vi "determine_harmonics.vi"(0 "FFT magnitude":cluster{"f0":dbl, "df":dbl, "magnitude":dbl[]}={"f0"=0.0, "df"=71.42857142857356, "magnitude"=array[7000 elements]}, 1 "FFT phase":cluster{"f0":dbl, "df":dbl, "phase":dbl[]}={"f0"=0.0, "df"=71.42857142857356, "phase"=array[7000 elements]}, 3 "TxRxParams":T1={"sample rate"=1000000.0, "Transmit frequency"=25000.0, "Transmit amplitude"=1.577, "sample rate digital out"=40000.0, "TX cycles"=600, "sample rate DAQ1"=1000000.0, "Receive frequency"=75000.0, "Receive range"=1.0, "TX harmonics"=[50000.0, 75000.0, 100000.0, 125000.0, 150000.0, 175000.0, 200000.0, 225000.0]} {"TX harmonics" format="%#_6p"; "Receive frequency" format="%#_6p"; "sample rate DAQ1" format="%#_6p"; "sample rate digital out" format="%#_6p"; "Transmit frequency" format="%#_6p"; "sample rate" format="%#_6p"}, 4 "TX harmonics mag baseline":dbl[](array[numeric])=[0.0, 0.0, 0.0, 0.0, 0.0, 0.0, 0.0, 0.0, 0.0, 0.0, 0.0], 5 "TX harmonics  phase baseline":dbl[](array[numeric])=[0.0, 0.0, 0.0, 0.0, 0.0, 0.0, 0.0, 0.0, 0.0, 0.0, 0.0], 6 "baseline phase":dbl, 7 "baseline magnitude":dbl) -> (12 "f0 phase":dbl=1.9394134400610221, 13 "f0 mag":dbl=0.024822285377457173, 14 "RX magnitude":dbl=0.0015696795969549263, 15 "RX phase":dbl=0.51499599210196, 17 "F3/F2":dbl, 18 "mag f2-f9":dbl[](array[numeric])=[0.07635364629802971, 0.0015696795969549263, 2.5850938198280388e-05, 3.5062095809530066e-05, 2.655041530081199e-05, 3.019279214108981e-05, 1.4173746366290001e-05, 4.367321701979328e-05], 19 "phase f2-f9":dbl[](array[numeric])=[2.093173382122955, 0.51499599210196, -2.573476238721069, 0.1764472036180968, -2.656638672525607, 2.555905242708201, -1.1093217629525705, -0.18697146017335703])   [LabVIEW 2021]
panel:
  out "TX harmonics":dbl[](array[numeric])=[50000.0, 75000.0, 100000.0, 125000.0, 150000.0, 175000.0, 200000.0, 225000.0] format="%#_6p"
  out "RxFreq":dbl=75000.0 format="%#_13g"
  out "TxFreq":dbl=25000.0 format="%#_13g"
  # "Inputs:"
  # "Keep default baseline value under all circumstances zero!!!!"
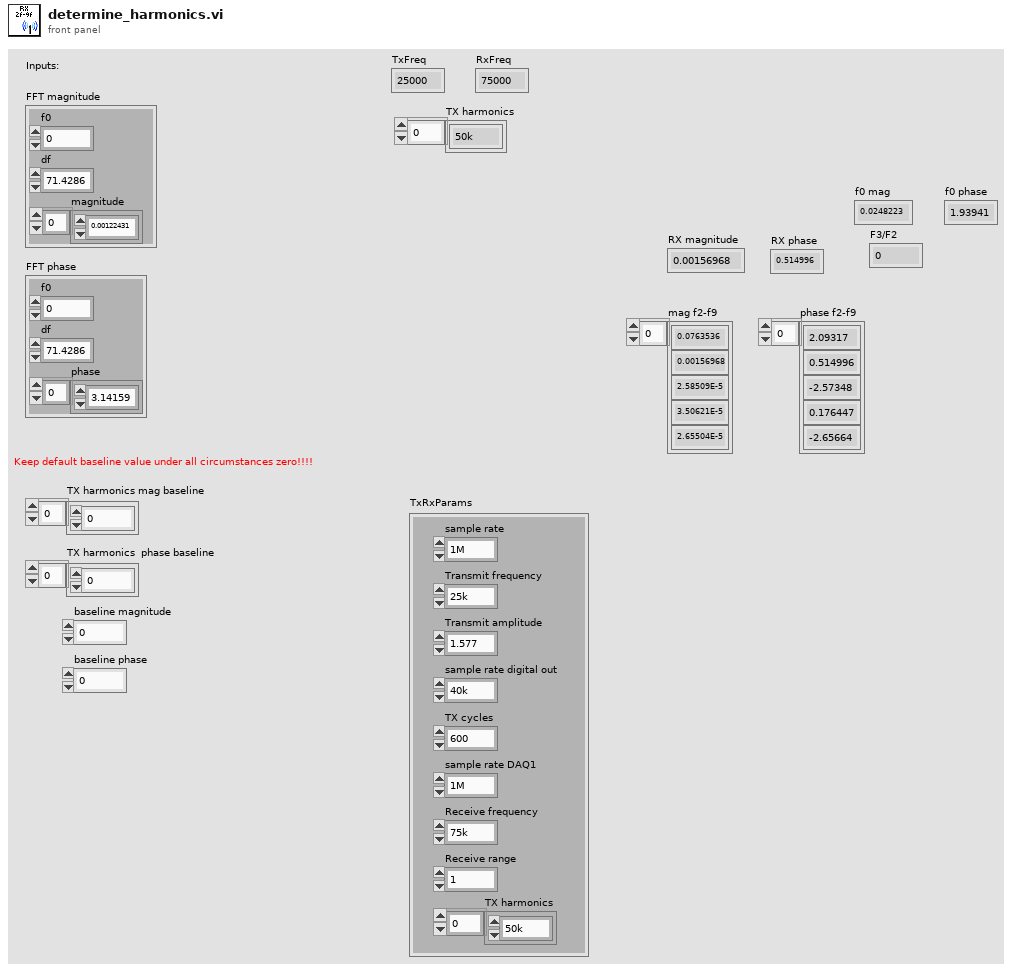
[diagram p1: front panel]
types:
  T1 = cluster{"sample rate":dbl, "Transmit frequency":dbl, "Transmit amplitude":dbl, "sample rate digital out":dbl, "TX cycles":i32, "sample rate DAQ1":dbl, "Receive frequency":dbl, "Receive range":dbl, "TX harmonics":dbl[]}
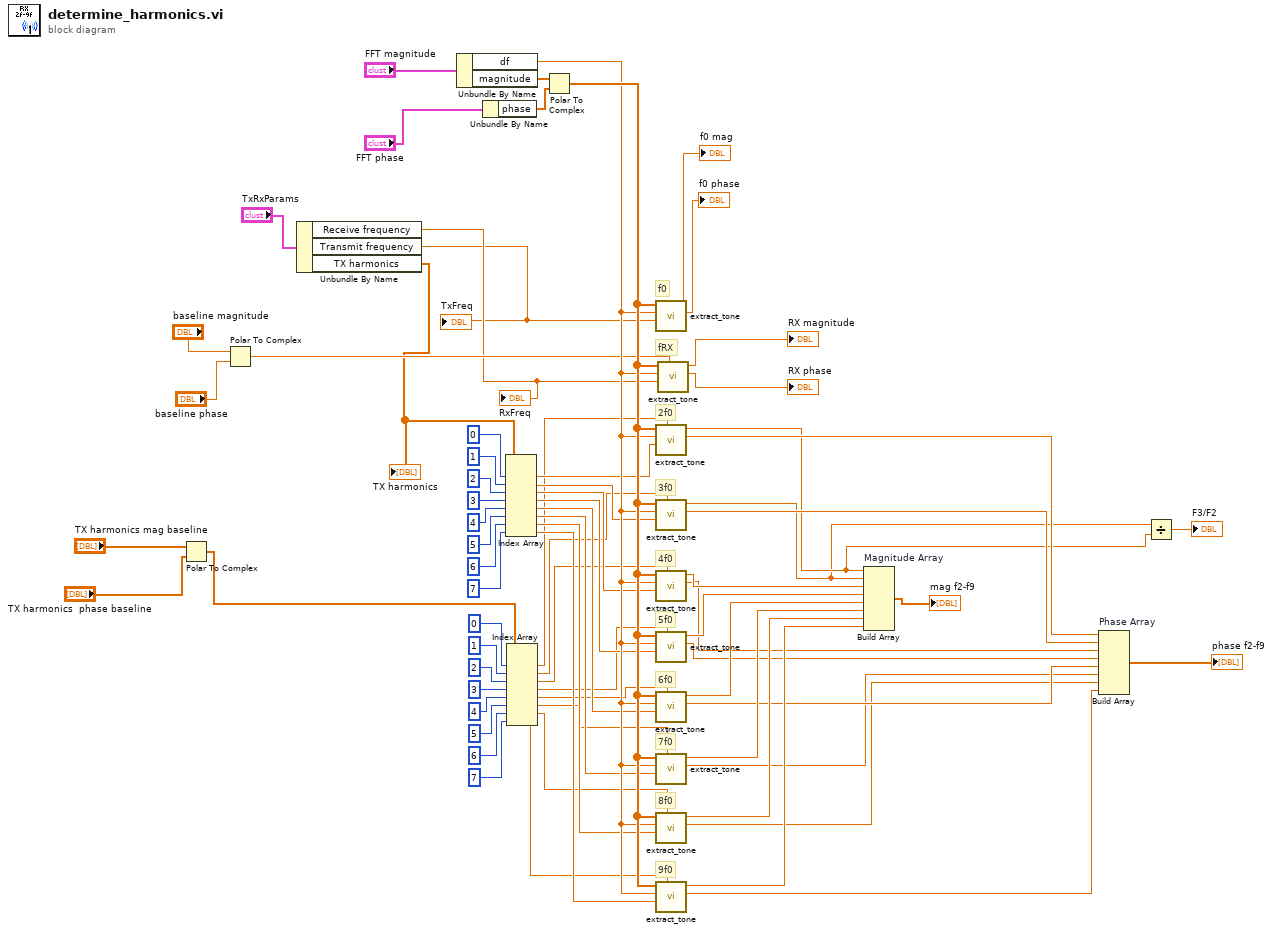
[diagram p0: block diagram]
diagram:
  # "fRX"
  # "9f0"
  # "8f0"
  # "7f0"
  # "6f0"
  # "5f0"
  # "4f0"
  # "3f0"
  # "2f0"
  # "f0"
  n1 = Polar To Complex(1:"TX harmonics  phase baseline", 2:"TX harmonics mag baseline") -> (0:w16:cdb[])
  n2 = Polar To Complex(1:"baseline phase", 2:"baseline magnitude") -> (0:w28:cdb)
  n3 = Unbundle By Name("TxRxParams") -> ("Receive frequency"=w6:dbl, "Transmit frequency"=w5:dbl, "TX harmonics"=w4:dbl[])
  "TxFreq" <- w5
  "RxFreq" <- w6
  "TX harmonics" <- w4
  n4 = Unbundle By Name("FFT magnitude") -> ("df"=w45:dbl, "magnitude"=w69:dbl[])
  n5 = Unbundle By Name("FFT phase") -> ("phase"=w68:dbl[])
  n6 = Index Array(array=w4, index #1=0 ("index"), index #2=1 ("index"), index #3=2 ("index"), index #4=3 ("index"), index #5=4 ("index"), index #6=5 ("index"), index #7=6 ("index"), index #8=7 ("index")) -> (element #1=w44:dbl, element #2=w35:dbl, element #3=w34:dbl, element #4=w33:dbl, element #5=w32:dbl, element #6=w31:dbl, element #7=w30:dbl, element #8=w29:dbl)
  n7 = Index Array(array=w16, index #1=0 ("index"), index #2=1 ("index"), index #3=2 ("index"), index #4=3 ("index"), index #5=4 ("index"), index #6=5 ("index"), index #7=6 ("index"), index #8=7 ("index")) -> (element #1=w15:cdb, element #2=w14:cdb, element #3=w13:cdb, element #4=w12:cdb, element #5=w11:cdb, element #6=w10:cdb, element #7=w9:cdb, element #8=w8:cdb)
  n8 = Polar To Complex(1:w68, 2:w69) -> (0:w46:cdb[])
  n9 = call "extract_tone.vi"("tone frequency [Hz]"=w5, "df"=w45, "complex fft"=w46) -> ("phase (rad)"=→"f0 phase":dbl, "amplitude"=→"f0 mag":dbl)  [unwired: 7 in]
  n10 = call "extract_tone.vi"("complex baseline"=w15, "tone frequency [Hz]"=w44, "df"=w45, "complex fft"=w46) -> ("phase (rad)"=w59:dbl, "amplitude"=w3:dbl)  [unwired: 6 in]
  n11 = call "extract_tone.vi"("complex baseline"=w14, "tone frequency [Hz]"=w35, "df"=w45, "complex fft"=w46) -> ("phase (rad)"=w50:dbl, "amplitude"=w2:dbl)  [unwired: 6 in]
  n12 = call "extract_tone.vi"("complex baseline"=w13, "tone frequency [Hz]"=w34, "df"=w45, "complex fft"=w46) -> ("phase (rad)"=w58:dbl, "amplitude"=w65:dbl)  [unwired: 6 in]
  n13 = call "extract_tone.vi"("complex baseline"=w12, "tone frequency [Hz]"=w33, "df"=w45, "complex fft"=w46) -> ("phase (rad)"=w57:dbl, "amplitude"=w64:dbl)  [unwired: 6 in]
  n14 = call "extract_tone.vi"("complex baseline"=w11, "tone frequency [Hz]"=w32, "df"=w45, "complex fft"=w46) -> ("phase (rad)"=w56:dbl, "amplitude"=w63:dbl)  [unwired: 6 in]
  n15 = call "extract_tone.vi"("complex baseline"=w10, "tone frequency [Hz]"=w31, "df"=w45, "complex fft"=w46) -> ("phase (rad)"=w55:dbl, "amplitude"=w62:dbl)  [unwired: 6 in]
  n16 = call "extract_tone.vi"("complex baseline"=w9, "tone frequency [Hz]"=w30, "df"=w45, "complex fft"=w46) -> ("phase (rad)"=w54:dbl, "amplitude"=w61:dbl)  [unwired: 6 in]
  n17 = call "extract_tone.vi"("complex baseline"=w8, "tone frequency [Hz]"=w29, "df"=w45, "complex fft"=w46) -> ("phase (rad)"=w53:dbl, "amplitude"=w60:dbl)  [unwired: 6 in]
  n18 = call "extract_tone.vi"("complex baseline"=w28, "tone frequency [Hz]"=w6, "df"=w45, "complex fft"=w46) -> ("phase (rad)"=→"RX phase":dbl, "amplitude"=→"RX magnitude":dbl)  [unwired: 6 in]
  n19 = Build Array "Magnitude Array"(w3, w2, w65, w64, w63, w62, w61, w60) -> (→"mag f2-f9":dbl[])
  n20 = Build Array "Phase Array"(w59, w50, w58, w57, w56, w55, w54, w53) -> (→"phase f2-f9":dbl[])
  n21 = Divide(x=w2, y=w3) -> (x/y=→"F3/F2":dbl)
